vi "Get External Channel Refs.vi"(8 "error in (no error)":errorcluster, 9 "Triggers":T2[](array[typedef]), 10 "Internal Trigger Refs":T1[](array[typedef]) format="%.0x", 11 "Device Ref in":T1 format="%.0x") -> (0 "error out":errorcluster, 2 "Refs":T3 {"Channels" format="%.0x"; "Triggers" format="%.0x"}, 3 "Item Ref out":T1 format="%.0x")   [LabVIEW 2019, in "Instrument Addon System Explorer.lvlib"]
uses:
  Instrument Addon System Explorer.lvlib
  <vilib>/NI VeriStand/Custom Device API/Custom Device Item Ref.ctl
  Addon Shared/Types/External Trigger Refs.ctl
  <vilib>/NI VeriStand/Custom Device API/Data Reference.ctl
  Addon Shared/Types/Trigger Parameters.ctl
  <vilib>/NI VeriStand/Custom Device API/Data Access Type.ctl
  <vilib>/NI VeriStand/Custom Device API/Custom Device API.lvlib
  <vilib>/NI VeriStand/Custom Device Tools/Custom Device Utility Library/Custom Device Utility Library.lvlib
  Addon Shared/Instrument Addon Shared.lvlib
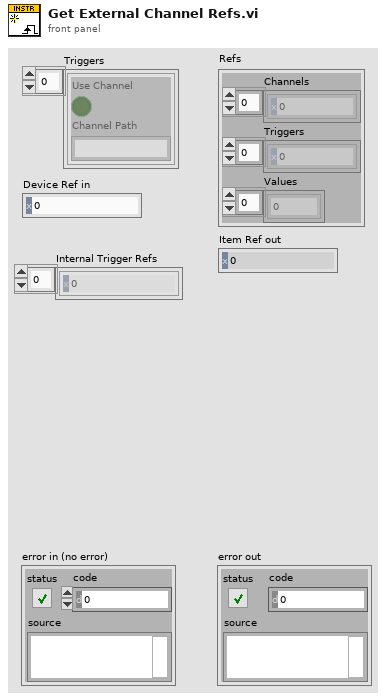
[diagram p1: front panel]
types:
  T1 = typedef "Custom Device API.lvlib/Custom Device Item Ref.ctl" = u64
  T2 = typedef "Instrument Addon Shared.lvlib/Trigger Parameters.ctl" = cluster{"Use Channel":bool, "Channel Path":string}
  T3 = typedef "Instrument Addon Shared.lvlib/External Trigger Refs.ctl" = cluster{"Channels":T4[], "Triggers":T4[], "Values":dbl[]}
  T4 = typedef "Custom Device API.lvlib/Data Reference.ctl" = i32
  T5 = typedef "Custom Device API.lvlib/Data Access Type.ctl" = enum16{"Read", "Write"}
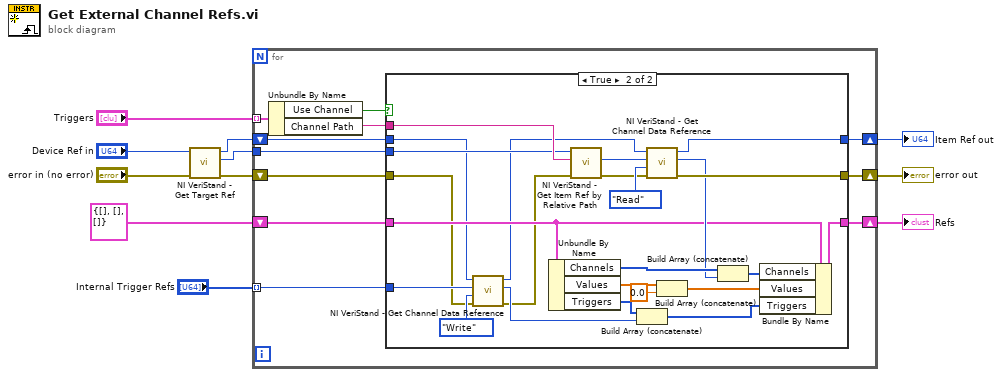
[diagram p0: block diagram]
diagram:
  n1 = call <vilib>:"NI VeriStand - Get Target Ref.vi"("error in"="error in (no error)", "Item Ref in"="Device Ref in") -> ("error out"=w4:errorcluster, "Target Ref"=w3:T1, "Item Ref out"=w5:T1)  [unwired: 6 in, 1 out]
  n2 = for {
    tunnel: "Triggers" -> [w22] mode=indexing
    tunnel: w3 -> [w21]
    shift-right: [w18] -> w9
    shift-left: w4 -> [w19]
    shift-right: [w16] -> w8
    shift-left: w5 -> [w17]
    shift-right: [w13] -> w6
    shift-left: T3 {"Channels"=[], "Triggers"=[], "Values"=[]} ("output cluster") -> [w14]
    tunnel: "Internal Trigger Refs" -> [w12] mode=indexing
    n3 = Unbundle By Name(w22) -> ("Use Channel"=w15:bool, "Channel Path"=w20:string)
    n4 = case shown="True" w15 {
      tunnel: w21 -> [_ w48]
      tunnel: w20 -> [_ w49]
      tunnel: w19 -> [w25 w27]
      tunnel: [w25 w43] -> w18
      tunnel: w17 -> [w24 w32]
      tunnel: [w24 w46] -> w16
      tunnel: w14 -> [w23 w38]
      tunnel: [w23 w35] -> w13
      tunnel: w12 -> [_ w28]
      frame False {
      }
      frame True {
        n5 = call <vilib>:"NI VeriStand - Get Channel Data Reference.vi"("error in (no error)"=w27, "Access"=Data_Access_Type."Write", "Channel Ref in"=w28, "Device Ref in"=w32) -> ("error out"=w26:errorcluster, "Channel Data Reference"=w30:T4, "Device Ref out"=w31:T1)  [unwired: 5 in]
        n6 = Unbundle By Name(w38) -> ("Channels"=w42:T4[], "Values"=w40:dbl[], "Triggers"=w33:T4[])
        n7 = call <vilib>:"NI VeriStand - Get Item Ref by Relative Path.vi"("error in"=w26, "Relative Item Path"=w49, "Section Ref in"=w48) -> ("error out"=w44:errorcluster, "Item Ref"=w47:T1)  [unwired: 5 in, 2 out]
        n8 = Build Array (concatenate)(w33, w30) -> (w34:T4[])
        n9 = call <vilib>:"NI VeriStand - Get Channel Data Reference.vi"("error in (no error)"=w44, "Access"=Data_Access_Type."Read", "Channel Ref in"=w47, "Device Ref in"=w31) -> ("error out"=w43:errorcluster, "Channel Data Reference"=w41:T4, "Device Ref out"=w46:T1)  [unwired: 5 in]
        n10 = Build Array (concatenate)(w40, 0.0) -> (w36:dbl[])
        n11 = Build Array (concatenate)(w42, w41) -> (w37:T4[])
        n12 = Bundle By Name(cluster=w38, "Channels"=w37, "Values"=w36, "Triggers"=w34) -> (w35:T3)
      }
    }
  }
  "error out" <- w9
  "Item Ref out" <- w8
  "Refs" <- w6
